vi "Pop Up.vi"(11 "Hello World Queue in":refnum<class "Hello World Queue.lvclass">) -> (3 "Hello World Queue out":refnum<class "Hello World Queue.lvclass">)   [LabVIEW 2021, in "Hello World Queue.lvlib" / "Hello World Queue.lvclass"]
uses:
  Hello World Queue.lvclass
  Hello World Queue.lvclass/Hello World Queue.ctl
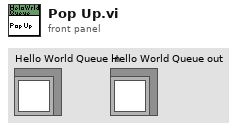
[diagram p1: front panel]
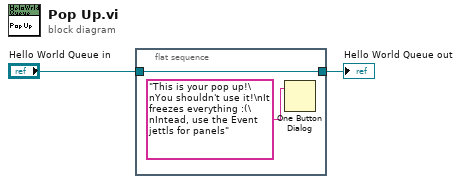
[diagram p0: block diagram]
diagram:
  n1 = flat-sequence {
    tunnel: "Hello World Queue in" -> [w3]
    tunnel: [w3] -> w1
    frame #0 {
      n2 = One Button Dialog(message="This is your pop up!\nYou shouldn't use it!\nIt freezes everything :(\nIntead, use the Event jettls for panels") -> ()  [unwired: 1 in, 1 out]
    }
  }
  "Hello World Queue out" <- w1
